vi "host_enable_read_target.vi"(8 "error in":errorcluster, 11 "enable read target?":bool) -> (0 "error out":errorcluster)   [LabVIEW 2021]
doc: "Stop reading a target on FPGA"
uses:
  core/host_global_vars.vi
  <vilib>/Utility/error.llb/Error Cluster From Error Code.vi
  <vilib>/rvi/errors/niLvFpgaAdjustHostInterfaceError.vi
  <vilib>/rvi/interface/nirviReadWriteControl/nirviReadWriteControl.xnode
  FPGA Bitfiles/openlabspm_FPGATarget_fpgamain_eo-gUZR5D1g.lvbitx
  fpga/fpga_main.vi
  NiFpgaLv.dll
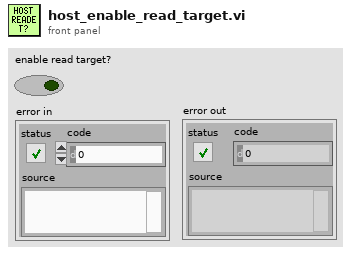
[diagram p1: front panel]
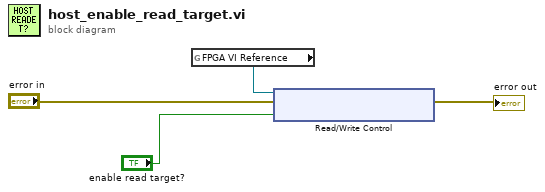
[diagram p0: block diagram]
diagram:
  n1 = global read "host_global_vars.vi" "FPGA VI Reference"() -> (w4:refnum<k20>)
  n2 = xnode "Read/Write Control"("FPGA VI Reference In"=w4, "error in"="error in", "enable read target"="enable read target?") -> ("error out"=→"error out":errorcluster)  [unwired: 1 out]
